vi "Recieve Request for Result.vi"(6 "Request time":timestamp, 8 "error in (no error)":errorcluster, 9 "Requestor":string, 10 "Requestee":string, 11 "RUS Measurement in":refnum<class "RUS Measurement.lvclass">) -> (0 "error out":errorcluster, 3 "RUS Measurement out":refnum<class "RUS Measurement.lvclass">)   [LabVIEW 2015, in "RUS Measurement.lvclass"]
uses:
  RUS Measurement.lvclass
  RUS Measurement.lvclass/RUS Measurement.ctl
  Mag Lab Root/Mag Lab Root.lvclass/Mag Lab Root.ctl
  <vilib>/ActorFramework/Actor/Actor.lvclass/Actor.ctl
  Mag Lab Root Messages/Recieve Request for Result Msg/Recieve Request for Result Msg.lvclass/Recieve Request for Result Msg.ctl
  <vilib>/ActorFramework/Message Enqueuer/Message Enqueuer.lvclass/Message Enqueuer.ctl
  Mag Lab Root/Read Name.vi
  Read RUS Instrument.vi
  Mag Lab Root/Write Request time.vi
  Mag Lab Root/Write Original requestor.vi
  <vilib>/ActorFramework/Message Enqueuer/Enqueue.vi
  <vilib>/ActorFramework/Message Priority Queue/Priority Enqueue.vi
  Mag Lab Root Messages/Recieve Request for Result Msg/Recieve Request for Result Msg.lvclass
  <vilib>/ActorFramework/Actor/Actor.lvclass
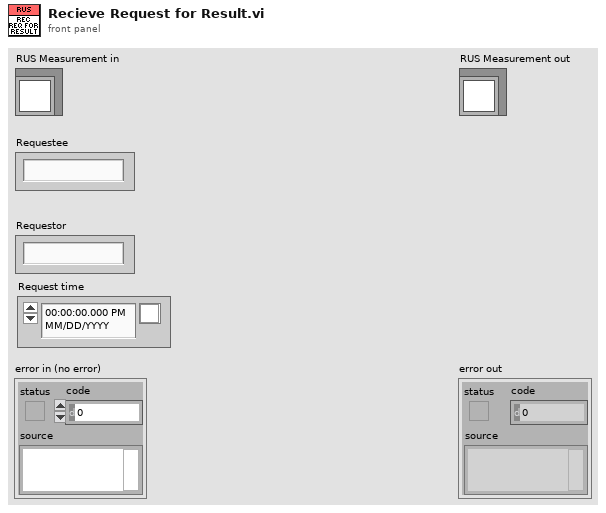
[diagram p1: front panel]
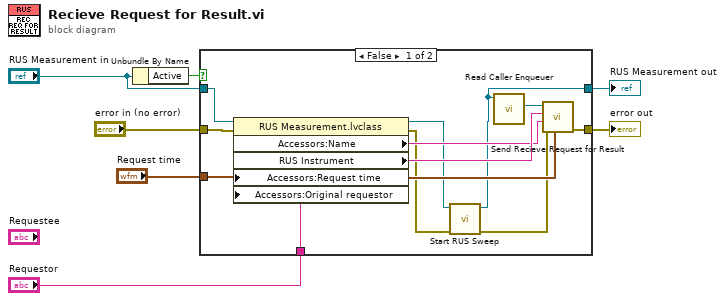
[diagram p0: block diagram]
diagram:
  n1 = Unbundle By Name("RUS Measurement in") -> ("Active"=w7:bool)
  n2 = case shown="False" w7 {
    tunnel: "RUS Measurement in" -> [w15 w21]
    tunnel: [w10 w21] -> w5
    tunnel: "Request time" -> [w13 _]
    tunnel: [w16 w20] -> w3
    tunnel: "error in (no error)" -> [w14 w20]
    tunnel: "Requestor" -> [w12 _]
    frame False {
      n3 = property class="RUS Measurement.lvclass"(reference=w15, error in=w14, "Accessors:Request time"=w13, "Accessors:Original requestor"=w12) -> (reference out=w11:refnum<class "RUS Measurement.lvclass">, error out=w9:errorcluster, "Accessors:Name"=w17:string, "RUS Instrument"=w18:string)
      n4 = call-dynamic "Start RUS Sweep.vi"("error in (no error)"=w9, "RUS Measurement in"=w11) -> ("error out"=w8:errorcluster, "RUS Measurement out"=w10:refnum<class "RUS Measurement.lvclass">)  [unwired: 8 in]
      n5 = call <vilib>:"Read Caller Enqueuer.vi"("Actor"=w10) -> ("Caller Enqueuer"=w19:refnum<class "Message Enqueuer.lvclass">)  [unwired: 10 in]
      n6 = call "Send Recieve Request for Result.vi"("Request time"=w13, "error in (no error)"=w8, "Requestor"=w17, "Requestee"=w18, "Message Enqueuer"=w19) -> ("error out"=w16:errorcluster)  [unwired: 5 in, 1 out]
    }
    frame True {
    }
  }
  "error out" <- w3
  "RUS Measurement out" <- w5
